vi "Send Stop Event.vi"(8 "error in (no error)":errorcluster, 11 "Subpanel Insertion.lvlib:Subpanel Inserter.lvclass":refnum<class "Subpanel Inserter.lvclass">) -> (0 "error out":errorcluster, 3 "Subpanel Inserter out":refnum<class "Subpanel Inserter.lvclass">)   [LabVIEW 2014, in "Subpanel Insertion.lvlib" / "Subpanel Inserter.lvclass"]
uses:
  Subpanel Inserter.lvclass
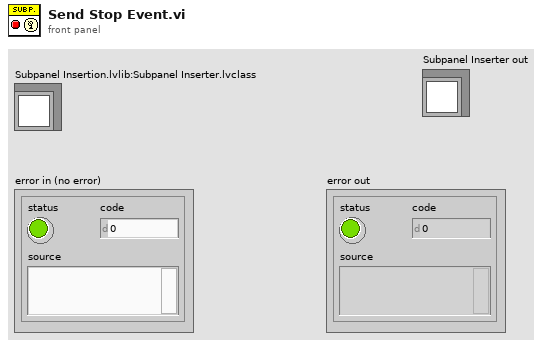
[diagram p1: front panel]
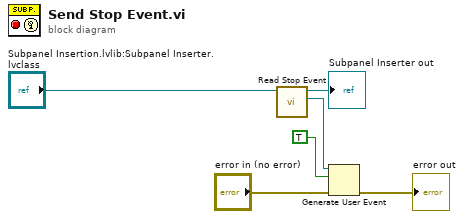
[diagram p0: block diagram]
diagram:
  n1 = call-dynamic "Read Stop Event.vi"("Subpanel Inserter in"="Subpanel Insertion.lvlib:Subpanel Inserter.lvclass") -> ("Stop Event"=w5:refnum<user-event>, "Subpanel Inserter out"=→"Subpanel Inserter out":refnum<class "Subpanel Inserter.lvclass">)  [unwired: 8 in, 1 out]
  n2 = Generate User Event(user event=w5, event data cluster=TRUE ("event data"), error in="error in (no error)") -> (error out=→"error out":errorcluster)  [unwired: 1 in, 1 out]
